vi "FisherPaykel Set Acceleration and Speed.vi"(0 "VISA Refnum in":refnum<visa-resource-name>, 1 "Debug":bool, 3 "Use GEA Inverter Output":bool, 5 "Spin Profile":T2={"Target Speed (RPM)"=23, "Acceleration Rate - (10 Slowest/1000 Fastest)"=20, "Running Time (s)"=20, "Direction (CW or CCW)"=""} {"Running Time (s)" step=1; "Acceleration Rate - (10 Slowest/1000 Fastest)" min=10 max=1000 step=1; "Target Speed (RPM)" min=23 max=1600 step=1}, 7 "GEA2 Reference In":refnum<k24>, 11 "Error In":errorcluster, 12 "Main Command":T4=">PS", 14 "GEA Inputs":T1={"Source"=228, "Destination"=35} {"Destination" format="%.0x"; "Source" format="%.0x"}) -> (4 "VISA resource name out":refnum<visa-resource-name>, 6 "Spin Profile Out":T2={"Target Speed (RPM)"=23, "Acceleration Rate - (10 Slowest/1000 Fastest)"=20, "Running Time (s)"=20, "Direction (CW or CCW)"=""} {"Running Time (s)" step=1; "Acceleration Rate - (10 Slowest/1000 Fastest)" min=10 max=1000 step=1; "Target Speed (RPM)" min=23 max=1600 step=1}, 8 "GEA2 Reference Out":refnum<k24>, 10 "Command (Debug)":string, 15 "Error Out":errorcluster)   [LabVIEW 2016]
uses:
  Type Definitions/Fisher Paykel Main Command.ctl
  Type Definitions/Fisher Paykel Motor Profile.ctl
  Type Definitions/FisherPaykel Direction CMD.ctl
  Trunk/Utility/LabVIEW GEA2 Toolkit v1.0.0.0/type defs/Source_Destination.ctl
  C:/Technology Lab/NI-2010/Trunk/Utility/LabVIEW GEA2 Toolkit v1.0.0.0/Appliance.NET/GeaCommunication.dll
  Trunk/Utility/LabVIEW GEA2 Toolkit v1.0.0.0/Appliance.NET/GeaCommunication.dll
  Trunk/Utility/LabVIEW GEA2 Toolkit v1.0.0.0/type defs/ERD Write Data In.ctl
  Trunk/Utility/LabVIEW GEA2 Toolkit v1.0.0.0/type defs/Data Type.ctl
  Trunk/Utility/LabVIEW GEA2 Toolkit v1.0.0.0/library/GEA2_Toolkit.lvlib
panel:
  # "Spin Profile Parameters"
  # "Spin Start Parameters"
  # "Spin Profile Parameters"
  # "Spin Start Parameters"
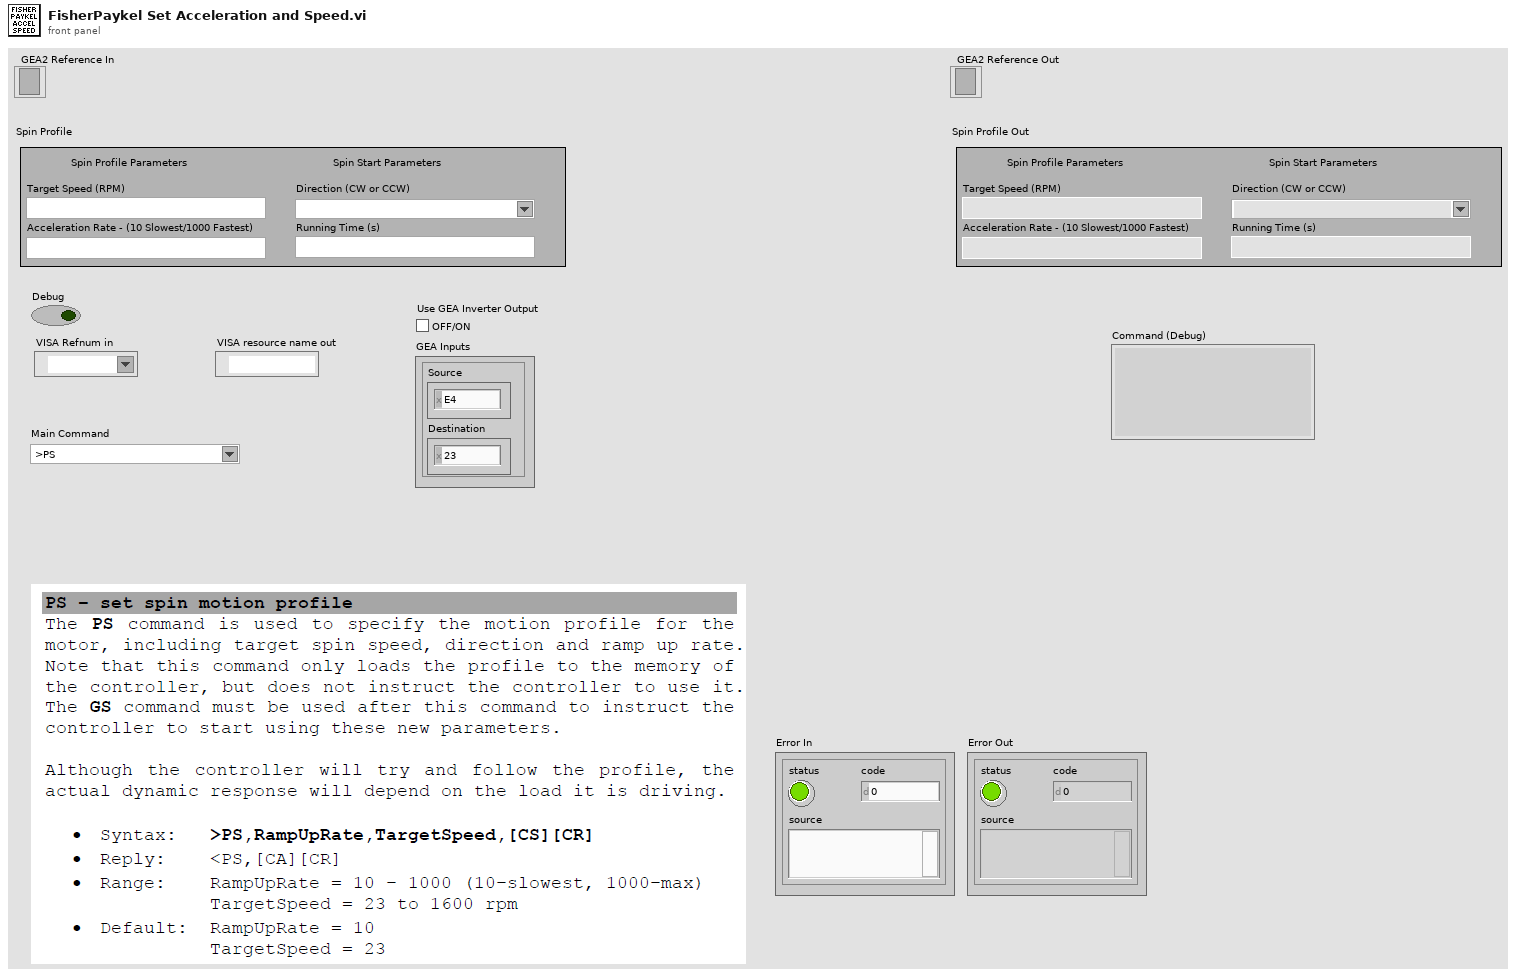
[diagram p1: front panel]
types:
  T1 = typedef "GEA2_Toolkit.lvlib/Source_Destination.ctl" = cluster{"Source":u8, "Destination":u8}
  T2 = typedef "Fisher Paykel Motor Profile.ctl" = cluster{"Target Speed (RPM)":u16, "Acceleration Rate - (10 Slowest/1000 Fastest)":u16, "Running Time (s)":u16, "Direction (CW or CCW)":T3}
  T3 = typedef "FisherPaykel Direction CMD.ctl" = string
  T4 = typedef "Fisher Paykel Main Command.ctl" = string
  T5 = typedef "GEA2_Toolkit.lvlib/ERD Write Data In.ctl" = cluster{"ERD Number":u16, "Data Type":T6, "Data":string}
  T6 = typedef "GEA2_Toolkit.lvlib/Data Type.ctl" = enum16{"string", "boolean", "uint8_t", "uint16_t", "uint32_t", "uint64_t"}
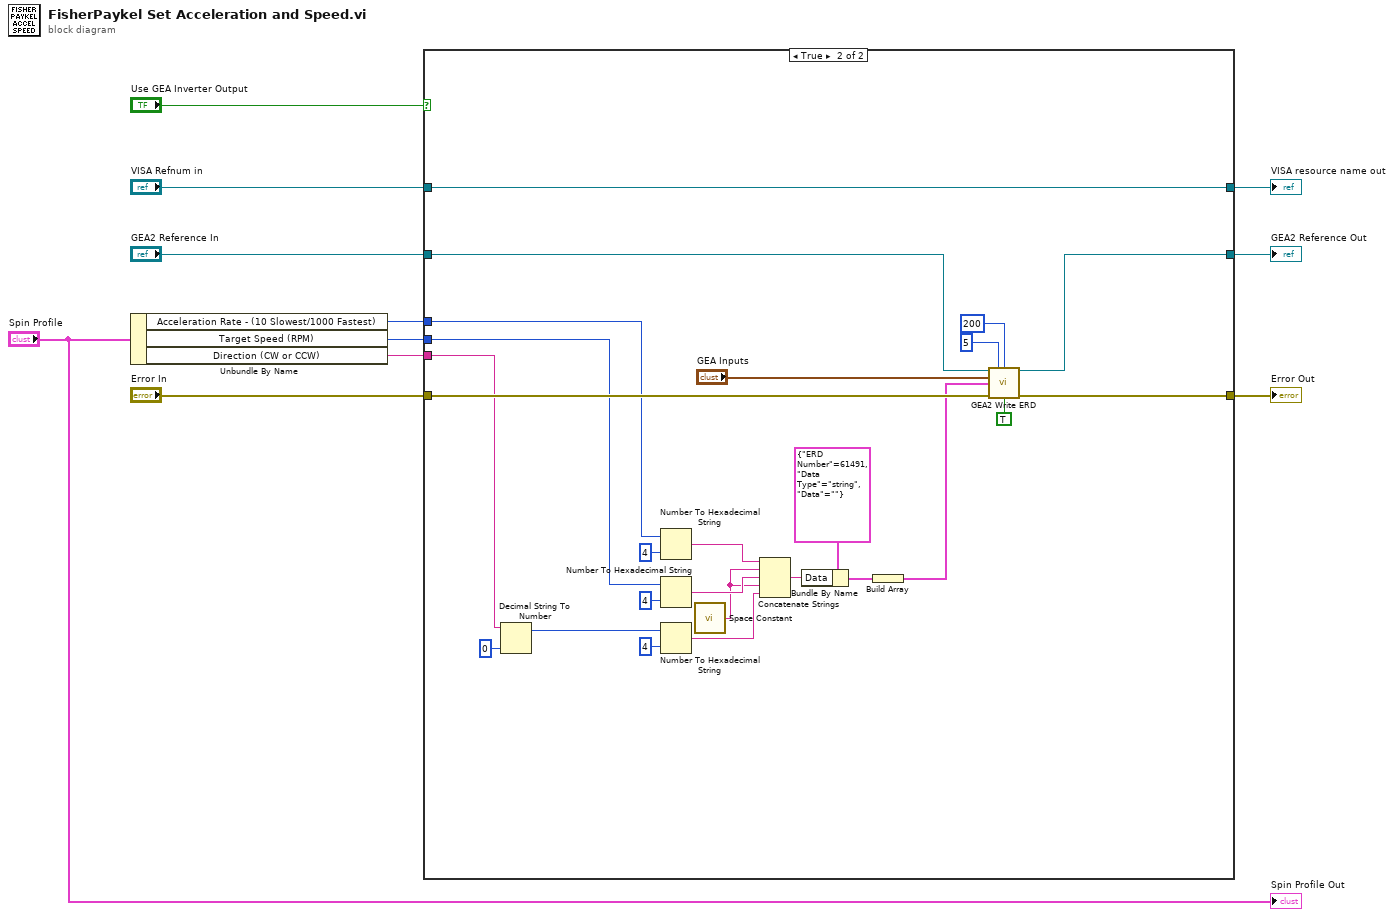
[diagram p0: block diagram]
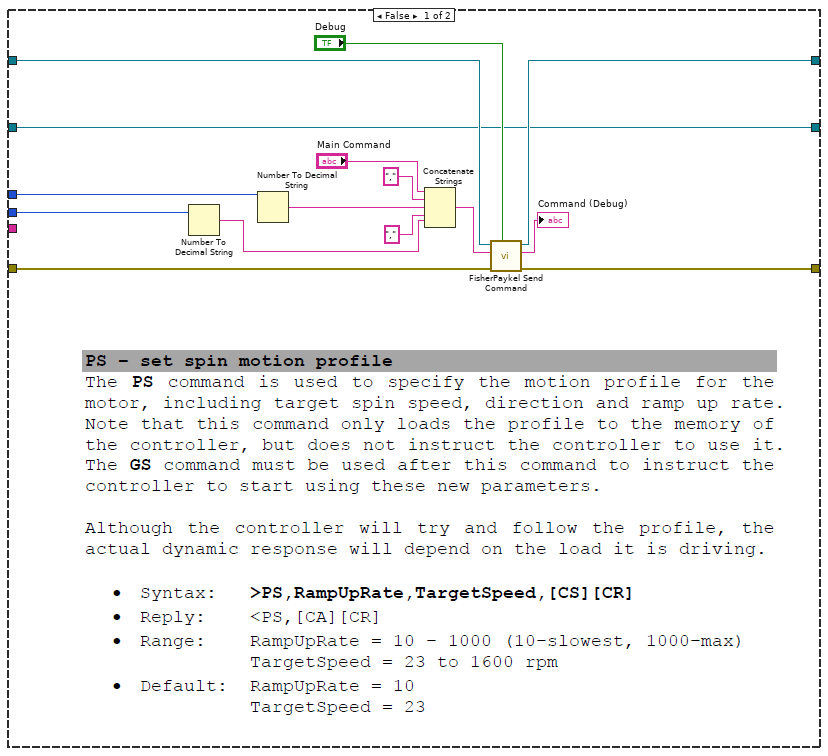
[diagram p2: hidden frame]
diagram:
  n1 = Unbundle By Name("Spin Profile") -> ("Acceleration Rate - (10 Slowest/1000 Fastest)"=w6:u16, "Target Speed (RPM)"=w5:u16, "Direction (CW or CCW)"=w1:T3)
  n2 = case shown="True" "Use GEA Inverter Output" {
    tunnel: "VISA Refnum in" -> [w26 w51]
    tunnel: "Error In" -> [w21 w46]
    tunnel: [w20 w51] -> w9
    tunnel: [w19 w45] -> w8
    tunnel: w6 -> [w16 w42]
    tunnel: w5 -> [w15 w41]
    tunnel: "GEA2 Reference In" -> [w12 w44]
    tunnel: [w12 w43] -> w2
    tunnel: w1 -> [_ w30]
    frame False {
      n3 = Number To Decimal String(number=w15) -> (decimal integer string=w14:string)  [unwired: 1 in]
      n4 = Number To Decimal String(number=w16) -> (decimal integer string=w13:string)  [unwired: 1 in]
      n5 = Concatenate Strings("Main Command", ",", w13, "," ("string"), w14) -> (w25:string)
      n6 = call "FisherPaykel Send Command.vi"("Debug"="Debug", "error in (no error)"=w21, "Send Command"=w25, "VISA Refnum in"=w26) -> ("error out"=w19:errorcluster, "Command (Debug)"=→"Command (Debug)":string, "VISA Refnum out"=w20:refnum<visa-resource-name>)  [unwired: 5 in]
    }
    frame True {
      n7 = Decimal String To Number(string=w30, default (0L)=u8 0 ("default (0 I32)")) -> (offset past number=w28:i32)  [unwired: 1 in, 1 out]
      n8 = Number To Hexadecimal String(1:i16 4 ("width (-)"), 2:w42) -> (0:w40:string)
      n9 = Number To Hexadecimal String(1:i16 4 ("width (-)"), 2:w41) -> (0:w39:string)
      n10 = Number To Hexadecimal String(1:i16 4 ("width (-)"), 2:w28) -> (0:w27:string)
      n11 = call <vilib>:"Space Constant.vi"() -> ("String"=w32:string)
      n12 = Concatenate Strings(w40, w32, w39, w32, w27) -> (w36:string)
      n13 = Bundle By Name(cluster=T5 {"ERD Number"=61491, "Data Type"=enum."string", "Data"=""} ("ERD Write Data In"), "Data"=w36) -> (w35:T5)
      n14 = Build Array(w35) -> (w38:T5[])
      n15 = call "GEA2 Write ERD.vi"("GEA2 Reference In"=w44, "Retry Count"=5, "Read Timeout (ms)"=u32 200, "GEA Inputs"="GEA Inputs", "Write ERD List"=w38, "Error In"=w46, "Verify ERD Response?"=TRUE) -> ("GEA2 Reference Out"=w43:refnum<k24>, "Error Out"=w45:errorcluster)  [unwired: 6 in, 1 out]
    }
  }
  "Error Out" <- w8
  "VISA resource name out" <- w9
  "GEA2 Reference Out" <- w2
  "Spin Profile Out" <- "Spin Profile"
